vi "Test WS Message Callback.vi"(7 "Owner":refnum<class>) -> (0 "error out":errorcluster)   [LabVIEW 2020]
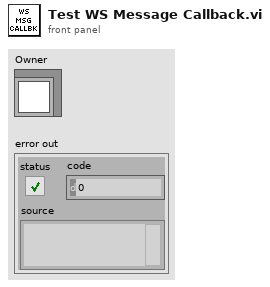
[diagram p1: front panel]
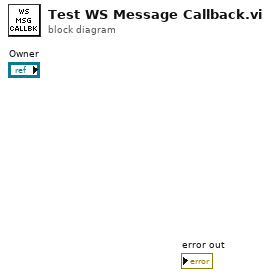
[diagram p0: block diagram]
diagram:
